vi "Initialize Instrument.vi"(8 "error in (no error)":errorcluster, 10 "Instrument Resource Name":string, 11 "Fluke DMM.lvclass in":refnum<class "Fluke DMM.lvclass">) -> (0 "error out":errorcluster, 3 "Fluke DMM.lvclass out":refnum<class "Fluke DMM.lvclass">)   [LabVIEW 2011, in "Fluke DMM.lvclass"]
uses:
  Fluke DMM.lvclass
  Fluke DMM.lvclass/Fluke DMM.ctl
  <instrlib>/Fluke 884X Series/Fluke 884X Series.lvlib
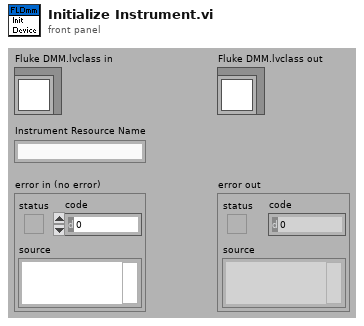
[diagram p1: front panel]
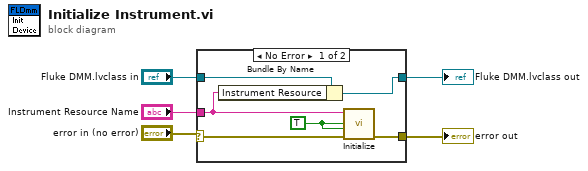
[diagram p0: block diagram]
diagram:
  n1 = case shown="No Error" "error in (no error)" {
    selector: "error in (no error)" -> [w10 w12]
    tunnel: "Fluke DMM.lvclass in" -> [w8 w13]
    tunnel: [w9 w12] -> w5
    tunnel: [w7 w13] -> w4
    tunnel: "Instrument Resource Name" -> [w6 _]
    frame No Error {
      w11 = TRUE ("ID Query? (T: Yes)")
      n2 = Bundle By Name(cluster=w8, "Instrument Resource"=w6) -> (w7:refnum<class "Fluke DMM.lvclass">)
      n3 = call <instrlib>:"Initialize.vi"("error in (no error)"=w10, "Reset (True)"=w11, "ID Query (True)"=w11, "VISA resource name"=w6) -> ("error out"=w9:errorcluster)  [unwired: 1 in, 6 out]
    }
    frame Error {
    }
  }
  "error out" <- w5
  "Fluke DMM.lvclass out" <- w4
